vi "FootStep_Demo_Cyclic.vi"() -> ()   [LabVIEW 2016]
uses:
  Foot_Demo_States.ctl
  Actuator/Controls/Command cluster.ctl
  Actuator/Controls/Command list.ctl
panel:
  out "status":bool
  in  "Positioning Threshold":dbl=0.1
  out "Waveform Chart":dbl(graph)
  in  "Speed Array":dbl[](array[numeric])=[20.0, 10.0] min=0.1 max=25.0 step=0.1
  in  "Position Array":dbl[](array[numeric])=[147.0, 130.0] min=0.1 max=150.0 step=0.1
  in  "Abort":bool
  in  "VISA resource name":refnum<visa-resource-name>="COM19"
  out "Device Information":string
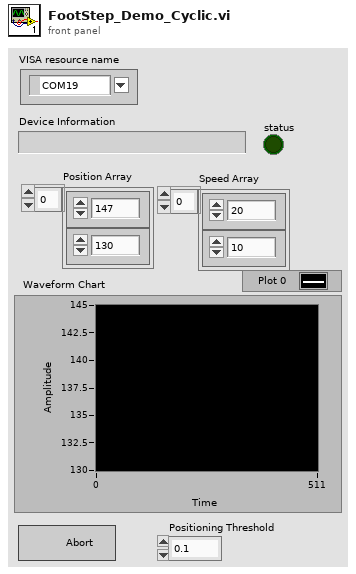
[diagram p1: front panel]
types:
  T1 = typedef "Command cluster.ctl" = cluster{"Command":T2, "data":variant}
  T2 = typedef "Command list.ctl" = enum16{"", "£nabort", "getaxisno", "£getserialno", "£nidentify", "&&£setnlimit", "&£nm", "&£snv", "&£speed", "£np", "£ncal"}
  T3 = typedef "Foot_Demo_States.ctl" = enum16{"Move", "Check Position", "Initialise"}
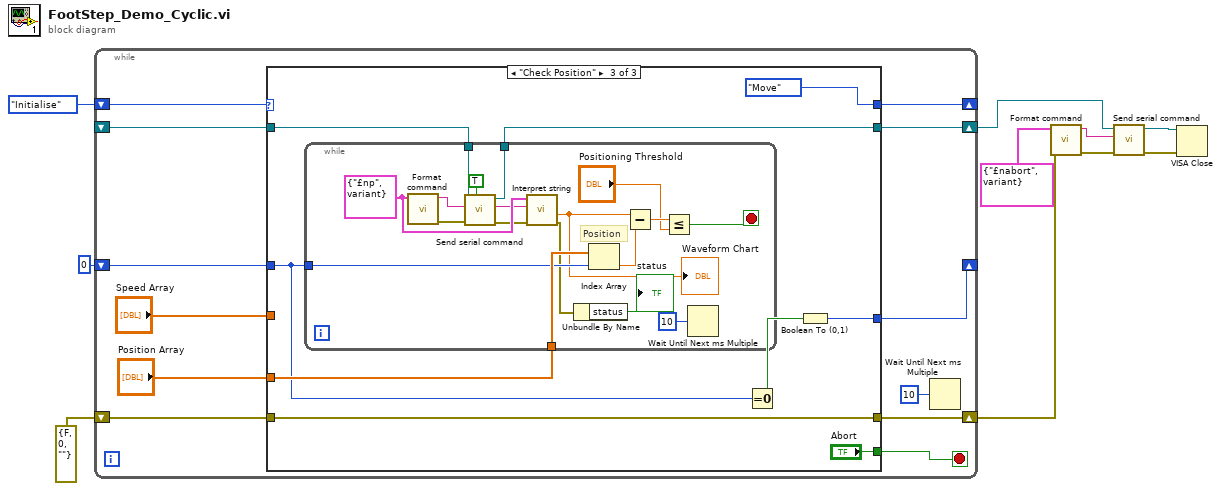
[diagram p0: block diagram]
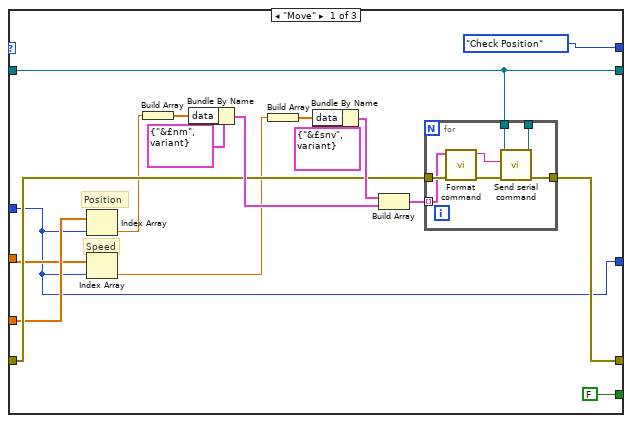
[diagram p2: hidden frame]
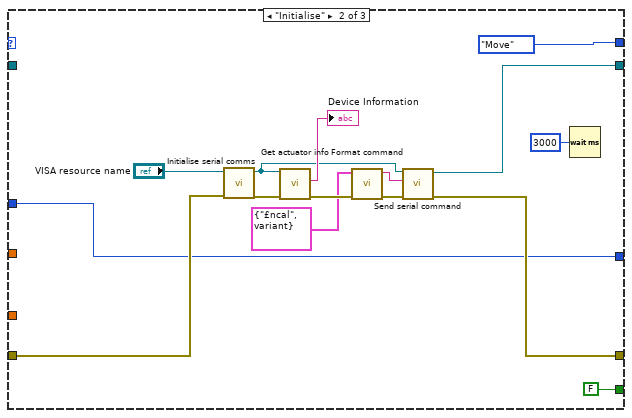
[diagram p3: hidden frame]
diagram:
  n1 = while {
    shift-right: [w19] -> _
    shift-left: Foot_Demo_States."Initialise" -> [w22]
    shift-right: [w21] -> w6
    shift-left: _ -> [w18]
    shift-right: [w16] -> w3
    shift-left: errorcluster {"status"=FALSE, "code"=0, "source"=""} ("error in (no error) 2") -> [w17]
    shift-right: [w11] -> _
    shift-left: u32 0 ("millisecond multiple") -> [w13]
    stop <- w20 stop-if-true
    n2 = case shown="\"Check Position\"" w22 {
      tunnel: [w23 w53 w68] -> w21
      tunnel: [FALSE ("Read?") FALSE ("Read?") "Abort"] -> w20
      tunnel: [Foot_Demo_States."Check Position" Foot_Demo_States."Move" Foot_Demo_States."Move"] -> w19
      tunnel: w18 -> [w23 _ w69]
      tunnel: w17 -> [w31 w51 w66]
      tunnel: [w32 w50 w66] -> w16
      tunnel: "Speed Array" -> [w27 _ _]
      tunnel: "Position Array" -> [w28 _ w67]
      tunnel: w13 -> [w25 w49 w65]
      tunnel: [w25 w49 w63] -> w11
      frame "Move" {
        # "Speed"
        # "Position"
        n3 = Index Array(array=w28, index=w25) -> (element=w29:dbl)
        n4 = Index Array(array=w27, index=w25) -> (element=w26:dbl)
        n5 = Build Array(w29) -> (w37:dbl[])
        n6 = Bundle By Name(cluster=T1 {"Command"=enum."&£nm", "data"=variant} ("Cluster"), "data"=w37) -> (w38:T1)
        n7 = Build Array(w26) -> (w39:dbl[])
        n8 = Bundle By Name(cluster=T1 {"Command"=enum."&£snv", "data"=variant} ("Cluster"), "data"=w39) -> (w36:T1)
        n9 = Build Array(w36, w38) -> (w30:T1[])
        n10 = for {
          tunnel: w23 -> [w44]
          tunnel: [w43] -> _
          tunnel: [w42] -> w32
          tunnel: w31 -> [w41]
          tunnel: w30 -> [w40] mode=indexing
          n11 = call "Format command.vi"("error in (no error)"=w41, "Cluster"=w40) -> ("error out"=w45:errorcluster, "String"=w46:string)  [unwired: 8 in]
          n12 = call "Send serial command.vi"("error IO"=w45, "Send string"=w46, "VISA resource name out"=w44) -> ("error out"=w42:errorcluster, "VISA Out"=w43:refnum<visa-resource-name>)  [unwired: 6 in, 1 out]
        }
      }
      frame "Initialise" {
        n13 = call "Initialise serial comms.vi"("error in (no error)"=w51, "VISA Refnum in"="VISA resource name") -> ("error out"=w54:errorcluster, "VISA Refnum out"=w59:refnum<visa-resource-name>)  [unwired: 7 in, 1 out]
        n14 = call "Get actuator info.vi"("error in (no error)"=w54, "VISA Refnum in"=w59) -> ("error out"=w56:errorcluster, "String"=→"Device Information":string)  [unwired: 7 in, 1 out]
        n15 = call "Format command.vi"("error in (no error)"=w56, "Cluster"=T1 {"Command"=enum."£ncal", "data"=variant}) -> ("error out"=w57:errorcluster, "String"=w58:string)  [unwired: 8 in]
        n16 = call "Send serial command.vi"("error IO"=w57, "Send string"=w58, "VISA resource name out"=w59) -> ("error out"=w50:errorcluster, "VISA Out"=w53:refnum<visa-resource-name>)  [unwired: 6 in, 1 out]
        n17 = Wait (ms)(milliseconds to wait=u32 3000) -> ()  [unwired: 1 out]
      }
      frame "Check Position" {
        n18 = while {
          tunnel: w69 -> [w82]
          tunnel: [w81] -> w68
          tunnel: w67 -> [w80]
          tunnel: w65 -> [w79]
          stop <- w75 stop-if-true
          w88 = T1 {"Command"=enum."£np", "data"=variant} ("Cluster")
          # "Position"
          n19 = call "Format command.vi"("Cluster"=w88) -> ("error out"=w86:errorcluster, "String"=w83:string)  [unwired: 9 in]
          n20 = call "Send serial command.vi"("Read?"=TRUE, "error IO"=w86, "Send string"=w83, "VISA resource name out"=w82) -> ("error out"=w87:errorcluster, "read string"=w85:string, "VISA Out"=w81:refnum<visa-resource-name>)  [unwired: 5 in]
          n21 = call "Interpret string.vi"("error in (no error)"=w87, "String"=w85, "Cluster"=w88) -> ("error out"=w72:errorcluster, "Numeric 2"=w74:dbl)  [unwired: 5 in, 2 out]
          "Waveform Chart" <- w74
          n22 = Unbundle By Name(w72) -> ("status"=→"status":bool)
          n23 = Index Array(array=w80, index=w79) -> (element=w77:dbl)
          n24 = Subtract(x=w74, y=w77) -> (x-y=w76:dbl)
          n25 = Less Or Equal?(x=w76, y="Positioning Threshold") -> (x <= y?=w75:bool)
          n26 = Wait Until Next ms Multiple(millisecond multiple=u32 10) -> ()  [unwired: 1 out]
        }
        n27 = Equal To 0?(x=w65) -> (x = 0?=w64:bool)
        n28 = Boolean To (0,1)(Boolean=w64) -> (0, 1=w63:i16)
      }
    }
    n29 = Wait Until Next ms Multiple(millisecond multiple=u32 10) -> ()  [unwired: 1 out]
  }
  n30 = call "Format command.vi"("error in (no error)"=w3, "Cluster"=T1 {"Command"=enum."£nabort", "data"=variant} ("Cluster 2")) -> ("error out"=w4:errorcluster, "String"=w7:string)  [unwired: 8 in]
  n31 = call "Send serial command.vi"("error IO"=w4, "Send string"=w7, "VISA resource name out"=w6) -> ("error out"=w1:errorcluster, "VISA Out"=w2:refnum<visa-resource-name>)  [unwired: 6 in, 1 out]
  n32 = VISA Close(VISA resource name=w2, error in (no error)=w1) -> ()  [unwired: 1 out]
